vi "Open Lidar.vi"(8 "error in (no error)":errorcluster, 10 "Lidar Number":i32) -> (0 "error out":errorcluster)   [LabVIEW 2016]
uses:
  Variables/MyRIO Lidar Class Data.vi
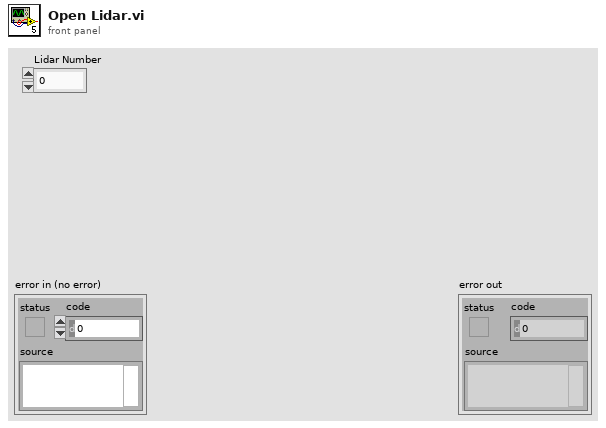
[diagram p1: front panel]
types:
  T1 = cluster{"Shared library path":path, "File Descriptor":i32}
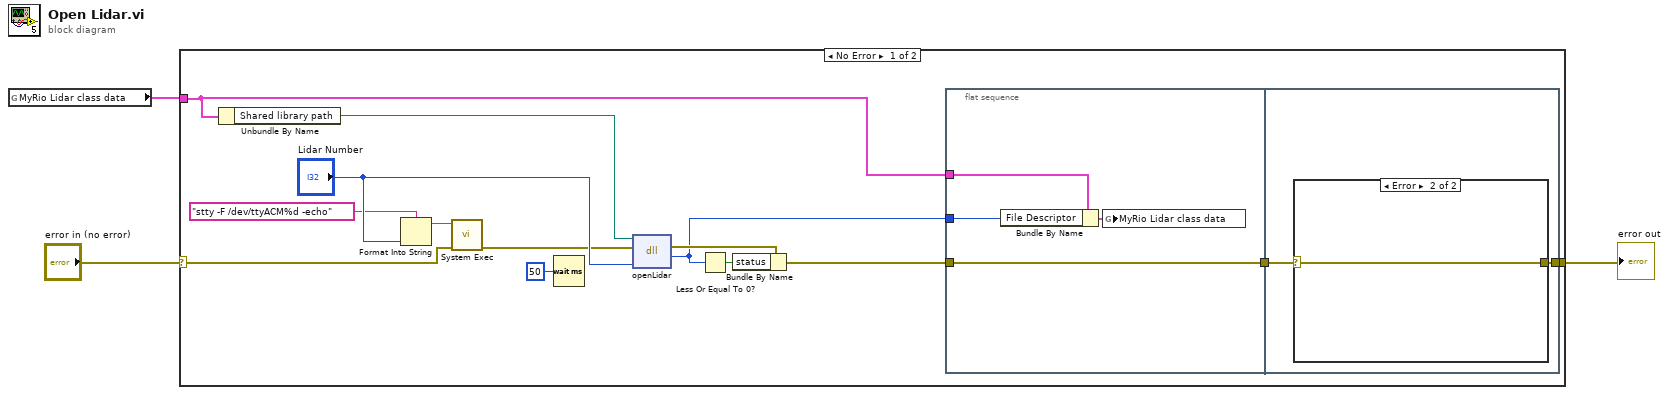
[diagram p0: block diagram]
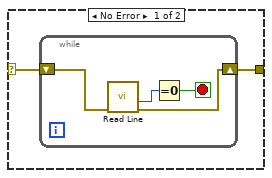
[diagram p2: hidden frame]
diagram:
  n1 = global read "MyRIO Lidar Class Data.vi" "MyRio Lidar class data"() -> (w1:T1)
  n2 = case shown="No Error" "error in (no error)" {
    selector: "error in (no error)" -> [w9 w31]
    tunnel: [w15 w31] -> w2
    tunnel: w1 -> [w4 _]
    frame No Error {
      n3 = Unbundle By Name(w4) -> ("Shared library path"=w14:path)
      n4 = Format Into String(format string="stty -F /dev/ttyACM%d -echo" ("command line"), "Lidar Number") -> (resulting string=w12:string)  [unwired: 2 in, 1 out]
      n5 = call <vilib>:"System Exec.vi"("error in (no error)"=w9, "command line"=w12) -> ("error out"=w8:errorcluster)  [unwired: 6 in, 3 out]
      n6 = Wait (ms)(milliseconds to wait=u32 50) -> ()  [unwired: 1 out]
      n7 = dll-call lib="?" fn="openLidar"(path in=w14, error in=w8, "lidarId"="Lidar Number") -> (error out=w7:errorcluster, "Return Value"=w5:i32)  [unwired: 2 in, 1 out]
      n8 = Less Or Equal To 0?(x=w5) -> (x <= 0?=w10:bool)
      n9 = Bundle By Name(cluster=w7, "status"=w10) -> (w17:errorcluster)
      n10 = flat-sequence {
        tunnel: w17 -> [w21]
        tunnel: [w21] -> w6
        tunnel: w4 -> [w19]
        tunnel: w5 -> [w18]
        tunnel: [w22] -> w15
        tunnel: w6 -> [w23]
        frame #0 {
          n11 = Bundle By Name(cluster=w19, "File Descriptor"=w18) -> (w20:T1)
          n12 = global write "MyRIO Lidar Class Data.vi" "MyRio Lidar class data"(w20) -> ()
        }
        frame #1 {
          n13 = case shown="Error" w23 {
            selector: w23 -> [w24 w30]
            tunnel: [w25 w30] -> w22
            frame No Error {
              n14 = while {
                shift-right: [w26] -> w25
                shift-left: w24 -> [w27]
                stop <- w28 stop-if-true
                n15 = call "Read Line.vi"("error in (no error)"=w27) -> ("error out"=w26:errorcluster, "Line length"=w29:i32)  [unwired: 8 in, 1 out]
                n16 = Equal To 0?(x=w29) -> (x = 0?=w28:bool)
              }
            }
            frame Error {
            }
          }
        }
      }
    }
    frame Error {
    }
  }
  "error out" <- w2
